vi "svacg_LimitTest Create Input Time Waveform based Limit.vi"(0 "waveform in":waveform(dbl), 1 "open interval? (T)":bool=TRUE, 5 "dt":dbl=1.0 format="%.2p", 7 "t0":timestamp, 9 "interpolation mode":u16(ring)=1 items=["coerce", "linear", "spline", "FIR filter"], 11 "error in":errorcluster, 12 "FIR filter specifications":T2={"alias rejection (dB)"=120.0, "normalized bandwidth"=0.4536} {"normalized bandwidth" format="%.4f"; "alias rejection (dB)" format="%.2f"}, 13 "Protection limits":T1={"Max oversampling ratio"=1024.0, "Max # output samples"=2097150}) -> (4 "limit waveform out":waveform(dbl), 10 "used t0":dbl format="%.2p", 14 "t0 adjusted warning":bool, 15 "error out":errorcluster)   [LabVIEW 2017]
uses:
  <vilib>/measure/NI_MAPro.lvlib
panel:
  # "open"
  # "closed"
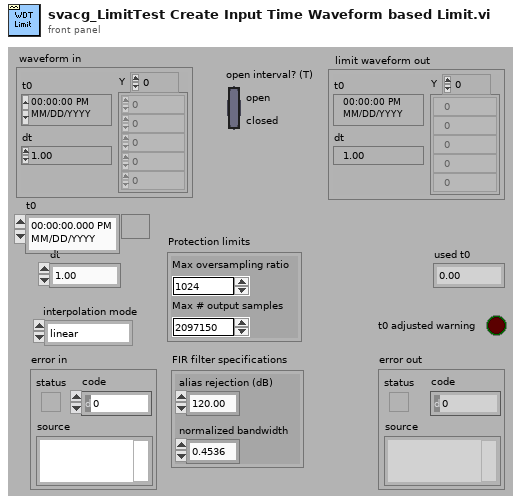
[diagram p1: front panel]
types:
  T1 = cluster{"Max oversampling ratio":dbl, "Max # output samples":i32}
  T2 = cluster{"alias rejection (dB)":dbl, "normalized bandwidth":dbl}
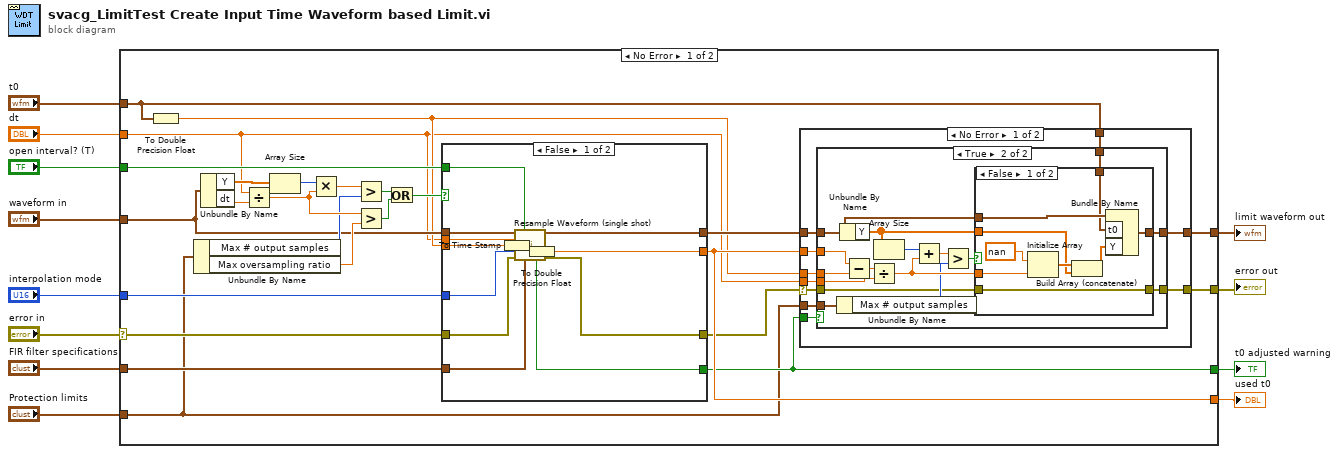
[diagram p0: block diagram]
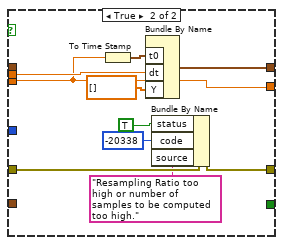
[diagram p2: hidden frame]
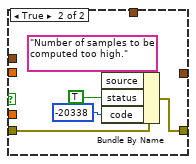
[diagram p4: hidden frame]
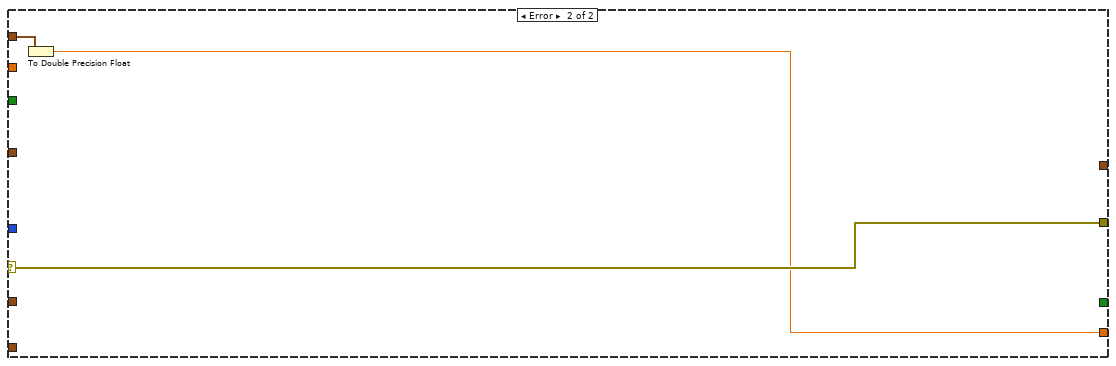
[diagram p6: hidden frame]
diagram:
  n1 = case shown="No Error" "error in" {
    selector: "error in" -> [w24 w106]
    tunnel: [w35 w106] -> w11
    tunnel: "waveform in" -> [w18 _]
    tunnel: "dt" -> [w13 _]
    tunnel: "t0" -> [w37 w105]
    tunnel: "Protection limits" -> [w15 _]
    tunnel: [w36 _] -> w6
    tunnel: "FIR filter specifications" -> [w23 _]
    tunnel: "interpolation mode" -> [w25 _]
    tunnel: "open interval? (T)" -> [w26 _]
    tunnel: [w21 w104] -> w2
    tunnel: [w19 _] -> w1
    frame No Error {
      n2 = To Double Precision Float(number=w37) -> (double precision float=w14:dbl)
      n3 = Unbundle By Name(w15) -> ("Max # output samples"=w27:i32, "Max oversampling ratio"=w28:dbl)
      n4 = Unbundle By Name(w18) -> ("Y"=w17:dbl[], "dt"=w16:dbl)
      n5 = Divide(x=w13, y=w16) -> (x/y=w33:dbl)
      n6 = Array Size(array=w17) -> (size(s)=w34:i32)
      n7 = Multiply(x=w34, y=w33) -> (x*y=w32:dbl)
      n8 = Greater?(x=w32, y=w27) -> (0:w31:bool)
      n9 = Greater?(x=w33, y=w28) -> (0:w30:bool)
      n10 = Or(x=w31, y=w30) -> (x .or. y?=w29:bool)
      n11 = case shown="False" w29 {
        tunnel: [w50 w57] -> w22
        tunnel: w24 -> [w49 w55]
        tunnel: [w48 w54] -> w20
        tunnel: w23 -> [w47 _]
        tunnel: w25 -> [w46 _]
        tunnel: w14 -> [w45 w56]
        tunnel: [w44 w56] -> w21
        tunnel: [w43 _] -> w19
        tunnel: w26 -> [w42 _]
        tunnel: w18 -> [w41 _]
        tunnel: w13 -> [w40 w59]
        frame False {
          n12 = To Time Stamp(1:w45) -> (0:w39:timestamp)
          n13 = call <vilib>:"Resample Waveform (single shot).vi"("waveform in"=w41, "open interval? (F)"=w42, "dt"=w40, "t0"=w39, "interpolation mode"=w46, "error in (no error)"=w49, "FIR filter specifications"=w47) -> ("resampled waveform out"=w50:waveform(dbl), "used t0"=w38:timestamp, "t0 adjusted warning"=w43:bool, "error out"=w48:errorcluster)  [unwired: 5 in]
          n14 = To Double Precision Float(number=w38) -> (double precision float=w44:dbl)
        }
        frame True {
          n15 = To Time Stamp(1:w56) -> (0:w60:timestamp)
          n16 = Bundle By Name("t0"=w60, "dt"=w59, "Y"=dbl[] []) -> (w57:waveform(dbl))  [unwired: 1 in]
          n17 = Bundle By Name(cluster=w55, "status"=TRUE, "code"=-20338, "source"="Resampling Ratio too high or number of samples to be computed too high.") -> (w54:errorcluster)
        }
      }
      n18 = case shown="No Error" w20 {
        selector: w20 -> [w61 w103]
        tunnel: w22 -> [w70 _]
        tunnel: w21 -> [w69 _]
        tunnel: w13 -> [w68 _]
        tunnel: w14 -> [w67 _]
        tunnel: w37 -> [w66 _]
        tunnel: w19 -> [w65 _]
        tunnel: [w64 _] -> w36
        tunnel: [w62 w103] -> w35
        tunnel: w15 -> [w63 _]
        frame No Error {
          n19 = case shown="True" w65 {
            tunnel: [w72 w86] -> w64
            tunnel: w70 -> [w72 w85]
            tunnel: w69 -> [_ w82]
            tunnel: w67 -> [_ w83]
            tunnel: w68 -> [_ w87]
            tunnel: w66 -> [_ w84]
            tunnel: w63 -> [_ w77]
            tunnel: [w71 w74] -> w62
            tunnel: w61 -> [w71 w73]
            frame False {
            }
            frame True {
              n20 = Unbundle By Name(w77) -> ("Max # output samples"=w76:i32)
              n21 = Unbundle By Name(w85) -> ("Y"=w81:dbl[])
              n22 = Subtract(x=w82, y=w83) -> (x-y=w88:dbl)
              n23 = Divide(x=w88, y=w87) -> (x/y=w79:dbl)
              n24 = Array Size(array=w81) -> (size(s)=w80:i32)
              n25 = Add(x=w80, y=w79) -> (x+y=w78:dbl)
              n26 = Greater?(x=w78, y=w76) -> (0:w75:bool)
              n27 = case shown="False" w75 {
                tunnel: [w95 _] -> w86
                tunnel: w85 -> [w94 _]
                tunnel: w84 -> [w92 _]
                tunnel: w81 -> [w91 _]
                tunnel: w79 -> [w90 _]
                tunnel: [w89 w99] -> w74
                tunnel: w73 -> [w89 w100]
                frame False {
                  n28 = Initialize Array(nan, w90) -> (w96:dbl[])
                  n29 = Build Array (concatenate)(w96, w91) -> (w93:dbl[])
                  n30 = Bundle By Name(cluster=w94, "t0"=w92, "Y"=w93) -> (w95:waveform(dbl))
                }
                frame True {
                  n31 = Bundle By Name(cluster=w100, "source"="Number of samples to be computed too high.", "status"=TRUE, "code"=-20338) -> (w99:errorcluster)
                }
              }
            }
          }
        }
        frame Error {
        }
      }
    }
    frame Error {
      n32 = To Double Precision Float(number=w105) -> (double precision float=w104:dbl)
    }
  }
  "limit waveform out" <- w6
  "error out" <- w11
  "t0 adjusted warning" <- w1
  "used t0" <- w2
